vi "_Update Experiment.vi"(4 "Expt#":i32, 5 "error in":errorcluster, 6 "Offset":u16, 7 "Expt":T1 {"Mass Range"."Resolution Type" items=["High/High", "Medium/Medium", "Low/Low", "High/Medium", "High/Low", "Medium/High", "Medium/Low", "Low/High", "Low/Medium"]}) -> (0 "error out":errorcluster, 1 "Next Offset":u16)   [LabVIEW 2012]
uses:
  Type/_RT Expt.ctl
  Type/_Run Mode.ctl
  Type/_RT Active Ch.ctl
  Type/_RT Mass Range.ctl
  Type/_RT Res Type.ctl
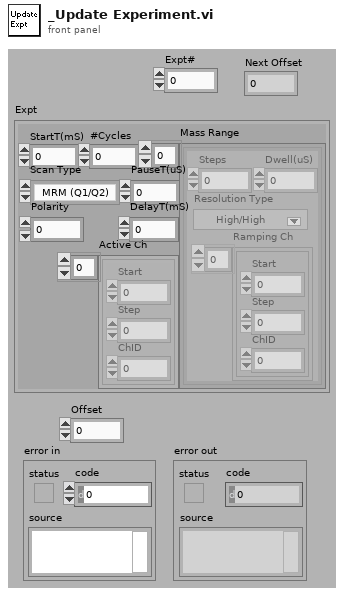
[diagram p1: front panel]
types:
  T1 = typedef "_RT Expt.ctl" = cluster{"StartT(mS)":i32, "#Cycles":i32, "Scan Type":T2, "PauseT(uS)":i32, "Polarity":u8, "DelayT(mS)":i32, "Active Ch":T3[], "Mass Range":T4[]}
  T2 = typedef "_Run Mode.ctl" = enum16{"MRM (Q1/Q2)", "Q1 Scan", "Q1 SRM", "Q2 Scan", "Q2 SRM", "Product Scan", "Precursor Scan", "Neutral Loss", "Neutral Gain"}
  T3 = typedef "_RT Active Ch.ctl" = cluster{"Start":i32, "Step":i32, "ChID":i32}
  T4 = typedef "_RT Mass Range.ctl" = cluster{"Steps":i32, "Dwell(uS)":i32, "Resolution Type":T5, "Ramping Ch":T3[]}
  T5 = typedef "_RT Res Type.ctl" = u16
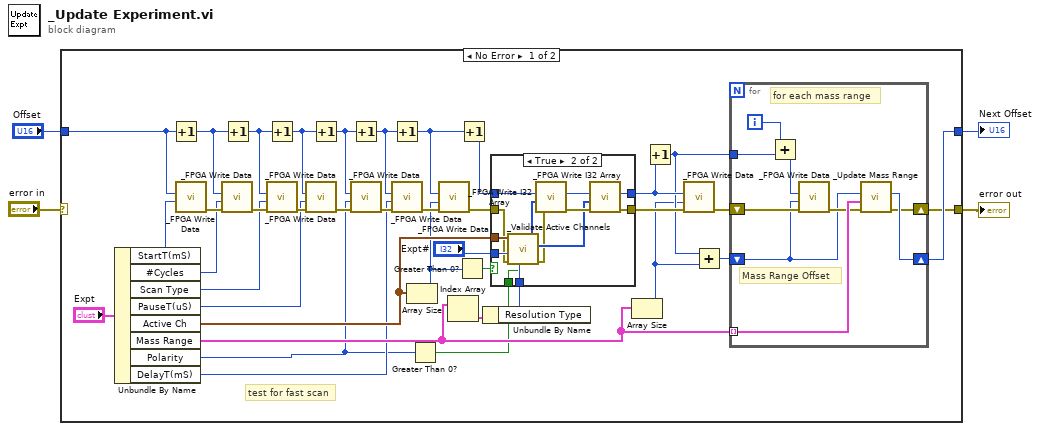
[diagram p0: block diagram]
diagram:
  n1 = case shown="No Error" "error in" {
    selector: "error in" -> [_ w68]
    tunnel: [w28 w68] -> w3
    tunnel: "Offset" -> [w30 w67]
    tunnel: [w29 w67] -> w1
    frame No Error {
      # "test for fast scan"
      n2 = Unbundle By Name("Expt") -> ("StartT(mS)"=w41:i32, "#Cycles"=w39:i32, "Scan Type"=w15:T2, "PauseT(uS)"=w7:i32, "Active Ch"=w24:T3[], "Mass Range"=w18:T4[], "Polarity"=w5:u8, "DelayT(mS)"=w6:i32)
      n3 = Increment(x=w30) -> (x+1=w38:u16)
      n4 = call "_FPGA Write Data.vi"("Data"=w41, "Address"=w30) -> ("error out"=w40:errorcluster)  [unwired: 4 in, 2 out]
      n5 = call "_FPGA Write Data.vi"("error in"=w40, "Data"=w39, "Address"=w38) -> ("error out"=w21:errorcluster)  [unwired: 3 in, 2 out]
      n6 = Increment(x=w38) -> (x+1=w20:u16)
      n7 = Increment(x=w20) -> (x+1=w12:u16)
      n8 = call "_FPGA Write Data.vi"("error in"=w21, "Data"=w15, "Address"=w20) -> ("error out"=w9:errorcluster)  [unwired: 3 in, 2 out]
      n9 = call "_FPGA Write Data.vi"("error in"=w9, "Data"=w7, "Address"=w12) -> ("error out"=w13:errorcluster)  [unwired: 3 in, 2 out]
      n10 = Increment(x=w12) -> (x+1=w11:u16)
      n11 = Increment(x=w11) -> (x+1=w10:u16)
      n12 = call "_FPGA Write Data.vi"("error in"=w13, "Data"=w5, "Address"=w11) -> ("error out"=w8:errorcluster)  [unwired: 3 in, 2 out]
      n13 = Increment(x=w10) -> (x+1=w22:u16)
      n14 = call "_FPGA Write Data.vi"("error in"=w8, "Data"=w6, "Address"=w10) -> ("error out"=w23:errorcluster)  [unwired: 3 in, 2 out]
      n15 = Array Size(array=w24) -> (size(s)=w19:i32)
      n16 = Greater Than 0?(x=w5) -> (x > 0?=w14:bool)
      n17 = call "_FPGA Write Data.vi"("error in"=w23, "Data"=w19, "Address"=w22) -> ("error out"=w36:errorcluster)  [unwired: 3 in, 2 out]
      n18 = Index Array(array=w18) -> (element=w17:T4)  [unwired: 1 in]
      n19 = Greater Than 0?(x=w19) -> (x > 0?=w34:bool)
      n20 = Increment(x=w22) -> (x+1=w37:u16)
      n21 = Unbundle By Name(w17) -> ("Resolution Type"=w16:T5)
      n22 = case shown="True" w34 {
        tunnel: w37 -> [w52 w66]
        tunnel: w36 -> [w53 w56]
        tunnel: [w53 w63] -> w35
        tunnel: [w52 w62] -> w31
        tunnel: w24 -> [_ w61]
        tunnel: "Expt#" -> [_ w58]
        tunnel: w16 -> [_ w57]
        tunnel: w14 -> [_ w54]
        frame False {
        }
        frame True {
          n23 = call "_Validate Active Channels.vi"("Negative (F)"=w54, "Resolution Type"=w57, "error in"=w56, "Expt#"=w58, "Active Ch"=w61) -> ("error out"=w55:errorcluster, "DAC Values"=w59:i32[], "Ch ID"=w60:i32[])  [unwired: 1 in, 1 out]
          n24 = call "_FPGA Write I32 Array.vi"("error in"=w55, "I32 Array"=w60, "Offset (0)"=w66) -> ("error out"=w65:errorcluster, "Next Offset"=w64:u16)  [unwired: 2 in, 1 out]
          n25 = call "_FPGA Write I32 Array.vi"("error in"=w65, "I32 Array"=w59, "Offset (0)"=w64) -> ("error out"=w63:errorcluster, "Next Offset"=w62:u16)  [unwired: 2 in, 1 out]
        }
      }
      n26 = Array Size(array=w18) -> (size(s)=w25:i32)
      n27 = Increment(x=w31) -> (x+1=w26:u16)
      n28 = call "_FPGA Write Data.vi"("error in"=w35, "Data"=w25, "Address"=w31) -> ("error out"=w33:errorcluster)  [unwired: 3 in, 2 out]
      n29 = Add(x=w26, y=w25) -> (x+y=w32:i32)
      n30 = for {
        shift-right: [w44] -> w28
        shift-left: w33 -> [w51]
        tunnel: w26 -> [w49]
        shift-right: [w45] -> w29
        shift-left: w32 -> [w46]
        tunnel: w18 -> [w48] mode=indexing
        i -> [w43]
        # "for each mass range"
        # "Mass Range Offset"
        n31 = Add(x=w43, y=w49) -> (x+y=w50:i32)
        n32 = call "_FPGA Write Data.vi"("error in"=w51, "Data"=w46, "Address"=w50) -> ("error out"=w47:errorcluster)  [unwired: 3 in, 2 out]
        n33 = call "_Update Mass Range.vi"("error in"=w47, "Mass Range"=w48, "Offset"=w46) -> ("error out"=w44:errorcluster, "Next Offset"=w45:u16)  [unwired: 1 in, 2 out]
      }
    }
    frame Error {
    }
  }
  "error out" <- w3
  "Next Offset" <- w1
